vi "set_sample_rate_record_length.vi"(8 "t max / us":dbl, 11 "Samples":i64) -> (0 "Min sample rate":dbl, 3 "Min record length":dbl)   [LabVIEW 2023]
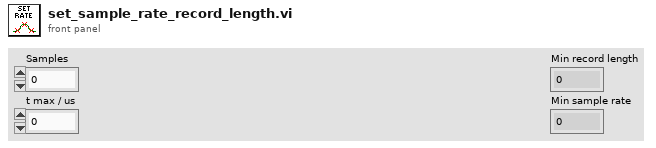
[diagram p1: front panel]
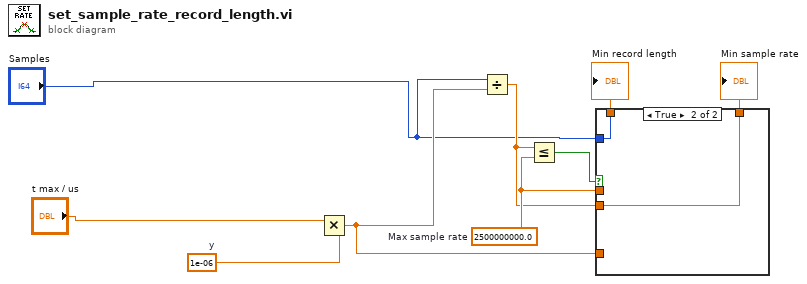
[diagram p0: block diagram]
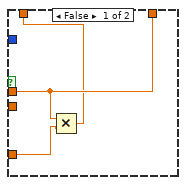
[diagram p2: hidden frame]
diagram:
  w7 = 2500000000.0  # Max sample rate
  w9 = 1e-06  # y
  n1 = Multiply(x="t max / us", y=w9) -> (x*y=w6:dbl)
  n2 = Divide(x="Samples", y=w6) -> (x/y=w5:dbl)
  n3 = Less Or Equal?(x=w5, y=w7) -> (x <= y?=w8:bool)
  n4 = case shown="True" w8 {
    tunnel: [w11 w14] -> w2
    tunnel: [w12 w13] -> w1
    tunnel: w7 -> [w12 _]
    tunnel: "Samples" -> [_ w14]
    tunnel: w5 -> [_ w13]
    tunnel: w6 -> [w10 _]
    frame False {
      n5 = Multiply(x=w12, y=w10) -> (x*y=w11:dbl)
    }
    frame True {
    }
  }
  "Min record length" <- w2
  "Min sample rate" <- w1
